vi "CNT Start.vi"(10 "ChannelMask":u8, 11 "DevIndex":i32) -> (3 "function return":i32)   [LabVIEW 2010, in "usb2cnt.lvlib"]
doc: "int WINAPI CNT_Start(int DevIndex, unsigned char ChannelMask);"
uses:
  usb2cnt.lvlib
  USB2XXX.dll
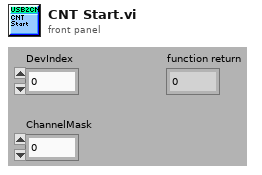
[diagram p1: front panel]
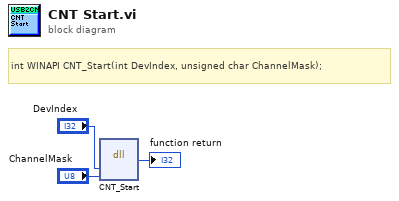
[diagram p0: block diagram]
diagram:
  # "int WINAPI CNT_Start(int DevIndex, unsigned char ChannelMask);"
  n1 = dll-call lib="G:/OtherWork/USB2XXX_Example/trunk/Labview/PublicFiles/usb2cnt/USB2XXX.*" fn="CNT_Start"("DevIndex"="DevIndex", "ChannelMask"="ChannelMask") -> (→"function return":i32)  [unwired: 5 in, 2 out]
